vi "Git current node.vi"(6 "ignore error (F)":bool, 8 "error in (no error)":errorcluster, 9 "Hash Char Length (6)":i32=6, 10 "Local Repo Path":path) -> (0 "error out":errorcluster, 1 "Current Branch":string, 2 "version string":string, 3 "Abreviated Hash":string)   [LabVIEW 2020]
doc: "Returns the current SVN revision and latest available SVN revision of the inputed vi or directory. Returns -1 if not versioned in SVN."
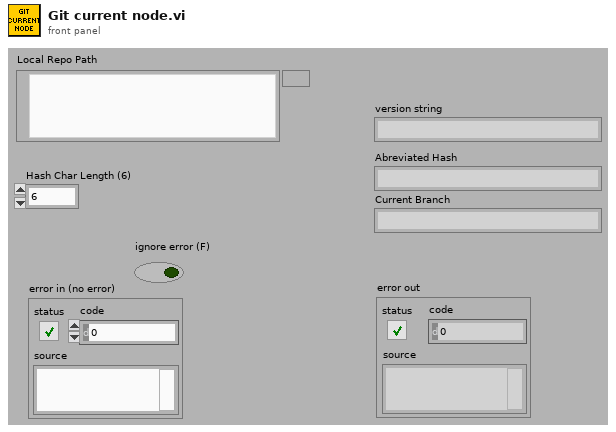
[diagram p1: front panel]
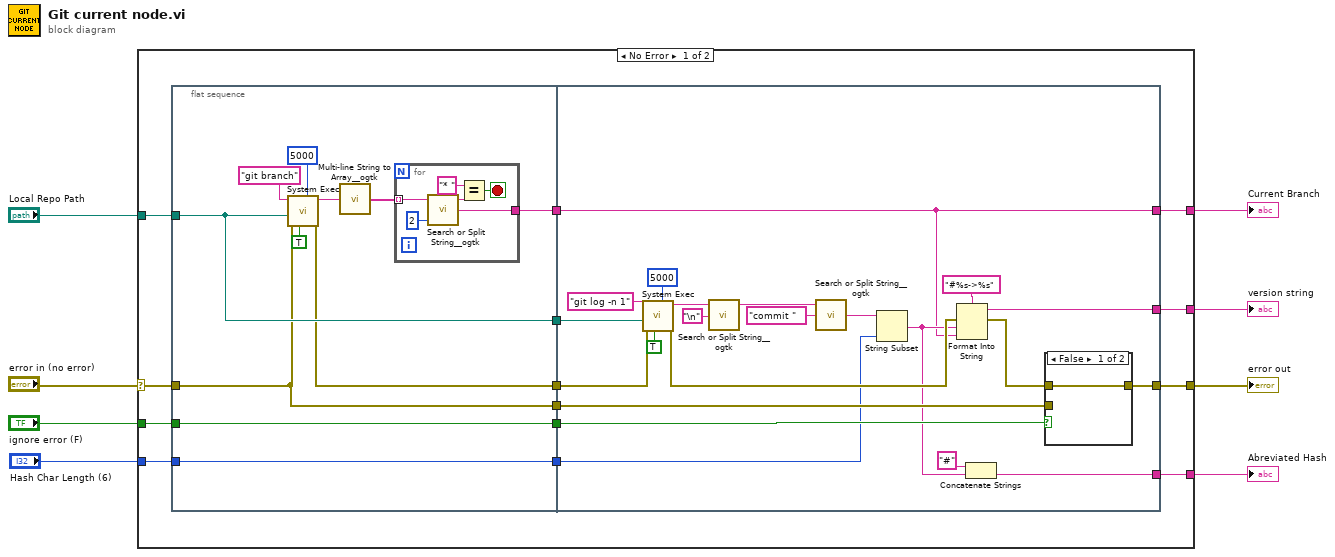
[diagram p0: block diagram]
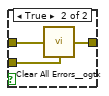
[diagram p2: hidden frame]
diagram:
  n1 = case shown="No Error" "error in (no error)" {
    selector: "error in (no error)" -> [w19 w66]
    tunnel: "Local Repo Path" -> [w20 _]
    tunnel: [w17 w66] -> w5
    tunnel: [w16 _] -> w6
    tunnel: "ignore error (F)" -> [w15 _]
    tunnel: [w12 _] -> w3
    tunnel: [w11 _] -> w2
    tunnel: "Hash Char Length (6)" -> [w9 _]
    frame No Error {
      n2 = flat-sequence {
        tunnel: w20 -> [w28]
        tunnel: [w28] -> w22
        tunnel: [w27] -> w21
        tunnel: w19 -> [w24]
        tunnel: [w26] -> w18
        tunnel: w15 -> [w25]
        tunnel: [w25] -> w14
        tunnel: [w24] -> w13
        tunnel: [w23] -> w10
        tunnel: w9 -> [w23]
        tunnel: w22 -> [w52]
        tunnel: w21 -> [w43]
        tunnel: w18 -> [w51]
        tunnel: [w49] -> w17
        tunnel: [w50] -> w16
        tunnel: w14 -> [w47]
        tunnel: w13 -> [w48]
        tunnel: [w42] -> w12
        tunnel: [w43] -> w11
        tunnel: w10 -> [w40]
        frame #0 {
          n3 = call <vilib>:"System Exec.vi"("expected output size  (4096)"=u32 5000, "run minimized? (F)"=TRUE, "error in (no error)"=w24, "working directory"=w28, "command line"="git branch") -> ("error out"=w26:errorcluster, "standard output"=w30:string)  [unwired: 3 in, 2 out]
          n4 = call <userlib>:"Multi-line String to Array__ogtk.vi"("string"=w30) -> ("lines"=w29:string[])
          n5 = for {
            tunnel: w29 -> [w38] mode=indexing
            tunnel: [w35] -> w27
            stop <- w36 stop-if-true
            n6 = call <userlib>:"Search or Split String__ogtk.vi"("offset (0)"=2, "string"=w38) -> ("substring after match"=w35:string, "substring before match"=w34:string)  [unwired: 1 in, 1 out]
            n7 = Equal?(x="* ", y=w34) -> (x = y?=w36:bool)
          }
        }
        frame #1 {
          n8 = call <vilib>:"System Exec.vi"("expected output size  (4096)"=u32 5000, "run minimized? (F)"=TRUE, "error in (no error)"=w51, "working directory"=w52, "command line"="git log -n 1") -> ("error out"=w46:errorcluster, "standard output"=w60:string)  [unwired: 3 in, 2 out]
          n9 = call <userlib>:"Search or Split String__ogtk.vi"("search string/char (-)"="\n", "string"=w60) -> ("substring before match"=w59:string)  [unwired: 1 in, 2 out]
          n10 = call <userlib>:"Search or Split String__ogtk.vi"("search string/char (-)"="commit ", "string"=w59) -> ("substring after match"=w61:string)  [unwired: 1 in, 2 out]
          n11 = String Subset(string=w61, length (rest)=w40) -> (substring=w44:string)  [unwired: 1 in]
          n12 = Format Into String(format string="#%s->%s", error in=w46, w44, w43) -> (resulting string=w50:string, error out=w45:errorcluster)  [unwired: 1 in]
          n13 = Concatenate Strings("#" ("string"), w44) -> (w42:string)
          n14 = case shown="False" w47 {
            tunnel: [w62 w65] -> w49
            tunnel: w48 -> [_ w64]
            tunnel: w45 -> [w62 w63]
            frame False {
            }
            frame True {
              n15 = call <userlib>:"Clear All Errors__ogtk.vi"("Upsteam Error (optional)"=w64, "Error In"=w63) -> ("Error Out"=w65:errorcluster)  [unwired: 2 in]
            }
          }
        }
      }
    }
    frame Error {
    }
  }
  "error out" <- w5
  "version string" <- w6
  "Abreviated Hash" <- w3
  "Current Branch" <- w2
